vi "ma_HasarrFIRSpecsChanged.vi"(4 "optional IIR filter specifications":T1(array[cluster]) {"SB Gain" format="%0.2f"; "PB Gain" format="%0.2f"}, 6 "IIR filter specs":T2(array[cluster]) {"Lower SB" format="%0.2p"; "Upper SB" format="%0.2p"; "Lower PB" format="%0.2p"; "Upper PB" format="%0.2p"}, 8 "error in (no error)":errorcluster, 10 "redesign filter":bool[](array[boolean])) -> (0 "error out":errorcluster, 3 "valsDifferent?":bool[](array[boolean]))   [LabVIEW 2020, in "NI_MAPro.lvlib"]
uses:
  NI_MAPro.lvlib
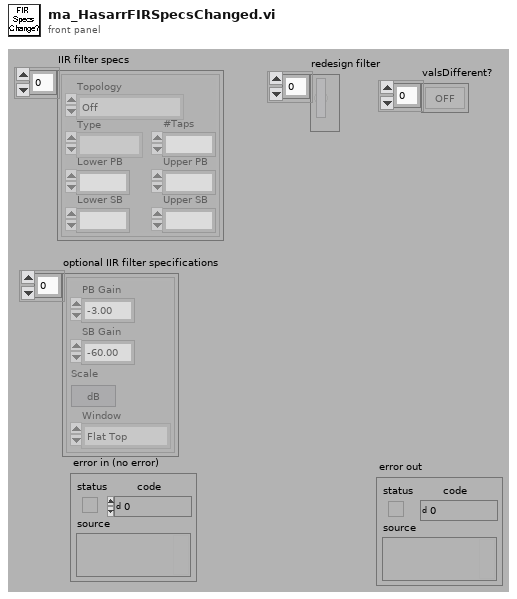
[diagram p1: front panel]
types:
  T1 = cluster{"PB Gain":dbl, "SB Gain":dbl, "Scale":bool, "Window":enum16{"None", "Hanning", "Hamming", "Triangular", "Blackman", "Exact Blackman", "Blackman-Harris", "Kaiser-Bessel", "Flat Top"}}[]
  T2 = cluster{"Topology":enum16{"Off", "FIR by Specification", "Equi-ripple FIR", "Windowed FIR"}, "Type":enum16{"Lowpass", "Highpass", "Bandpass", "Bandstop"}, "#Taps":i32, "Lower PB":dbl, "Upper PB":dbl, "Lower SB":dbl, "Upper SB":dbl}[]
  T3 = cluster{"PB Gain":dbl, "SB Gain":dbl, "Scale":bool, "Window":enum16{"None", "Hanning", "Hamming", "Triangular", "Blackman", "Exact Blackman", "Blackman-Harris", "Kaiser-Bessel", "Flat Top"}}
  T4 = cluster{"Topology":enum16{"Off", "FIR by Specification", "Equi-ripple FIR", "Windowed FIR"}, "Type":enum16{"Lowpass", "Highpass", "Bandpass", "Bandstop"}, "#Taps":i32, "Lower PB":dbl, "Upper PB":dbl, "Lower SB":dbl, "Upper SB":dbl}
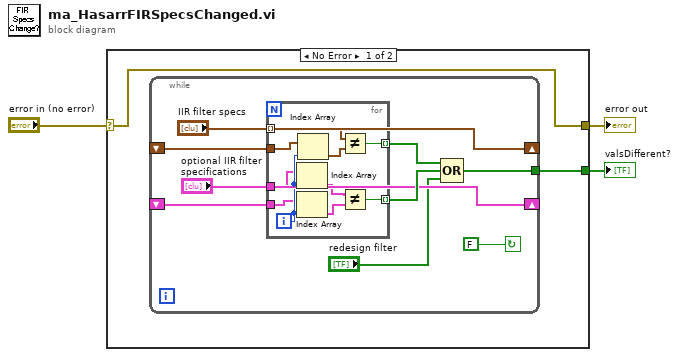
[diagram p0: block diagram]
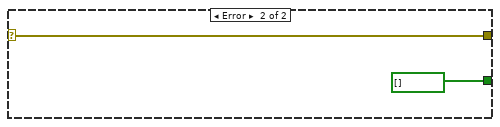
[diagram p2: hidden frame]
diagram:
  n1 = case shown="No Error" "error in (no error)" {
    selector: "error in (no error)" -> [w4 w26]
    tunnel: [w5 bool[] [] ("Array Constant")] -> w1
    tunnel: [w4 w26] -> w2
    frame No Error {
      n2 = while {
        shift-left: _ -> [w13]
        shift-right: ["optional IIR filter specifications"] -> _
        tunnel: [w9] -> w5
        shift-left: _ -> [w12]
        shift-right: ["IIR filter specs"] -> _
        stop <- FALSE continue-if-true
        n3 = for {
          tunnel: w13 -> [w20]
          tunnel: w12 -> [w15]
          tunnel: [w24] -> w11 mode=indexing
          tunnel: [w23] -> w10 mode=indexing
          tunnel: "IIR filter specs" -> [w22] mode=indexing
          tunnel: "optional IIR filter specifications" -> [w17]
          i -> [w21]
          n4 = Index Array(array=w17, index=w21) -> (element=w18:T3)
          n5 = Index Array(array=w20, index=w21) -> (element=w19:T3)
          n6 = Index Array(array=w15, index=w21) -> (element=w16:T4)
          n7 = Not Equal?(x=w22, y=w16) -> (x != y?=w24:bool)
          n8 = Not Equal?(x=w18, y=w19) -> (x != y?=w23:bool)
        }
        n9 = Compound Arithmetic op=OR(w11, w10, "redesign filter") -> (w9:bool[])
      }
    }
    frame Error {
    }
  }
  "error out" <- w2
  "valsDifferent?" <- w1
